vi "Enum.vi"() -> ()   [LabVIEW 2021]
uses:
  <vilib>/measure/NI_MABase.lvlib
panel:
  in  "Signal Type":enum16{"Sine", "Trin", "Squa", "Swa"}(ring)
  in  "Amplitude":dbl(knob) scale=0.0..10.0
  in  "Frequency":dbl(knob) scale=0.0..100.0
  out "Waveform Graph":waveform(dbl)(graph)
  in  "Stop":bool
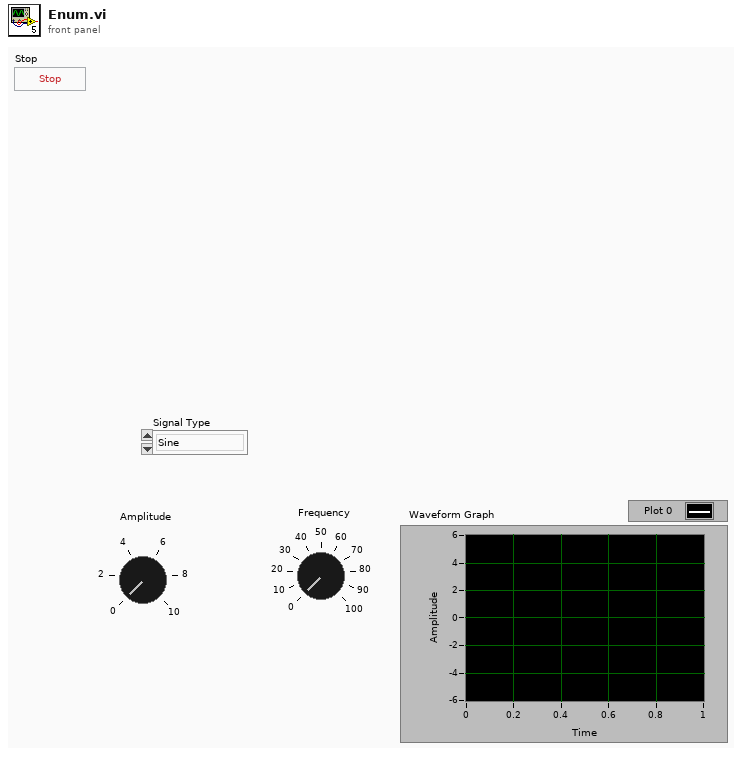
[diagram p1: front panel]
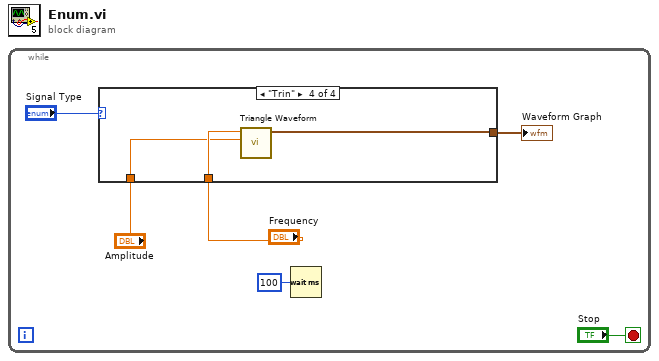
[diagram p0: block diagram]
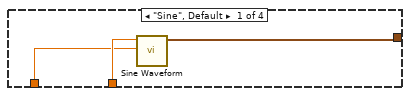
[diagram p2: hidden frame]
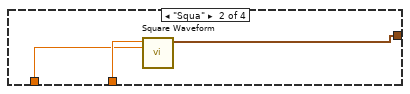
[diagram p3: hidden frame]
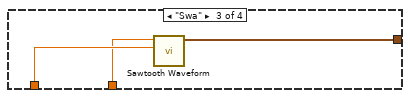
[diagram p4: hidden frame]
diagram:
  n1 = while {
    stop <- "Stop" stop-if-true
    n2 = case shown="\"Trin\"" "Signal Type" {
      tunnel: "Frequency" -> [w9 w12 w14 w18]
      tunnel: "Amplitude" -> [w8 w11 w15 w17]
      tunnel: [w7 w10 w13 w16] -> w3
      frame "Sine", Default {
        n3 = call <vilib>:"Sine Waveform.vi"("amplitude"=w8, "frequency"=w9) -> ("signal out"=w7:waveform(dbl))  [unwired: 8 in, 1 out]
      }
      frame "Squa" {
        n4 = call <vilib>:"Square Waveform.vi"("amplitude"=w11, "frequency"=w12) -> ("signal out"=w10:waveform(dbl))  [unwired: 8 in, 1 out]
      }
      frame "Swa" {
        n5 = call <vilib>:"Sawtooth Waveform.vi"("amplitude"=w15, "frequency"=w14) -> ("signal out"=w13:waveform(dbl))  [unwired: 8 in, 1 out]
      }
      frame "Trin" {
        n6 = call <vilib>:"Triangle Waveform.vi"("amplitude"=w17, "frequency"=w18) -> ("signal out"=w16:waveform(dbl))  [unwired: 8 in, 1 out]
      }
    }
    "Waveform Graph" <- w3
    n7 = Wait (ms)(milliseconds to wait=u32 100) -> ()  [unwired: 1 out]
  }
